vi "kvCanAccept.vi"(2 "error in (no error)":errorcluster, 3 "Accept Flag":i32(ring)=3 items=["Reserve 0", "Reserve 1", "Reserve 2", "Set Standard Code", "Set Standard Mask", "Set Extended Code", "Set Extended Mask"], 4 "Envelope Mask or Code":u32, 5 "Channel Handle (input only)":i32) -> (0 "error out":errorcluster, 1 "Channel Handle (ouput only)":i32)   [LabVIEW 2022 SP3]
doc: "This routine sets the message acceptance filters on a CAN channel."
uses:
  canlib32.dll
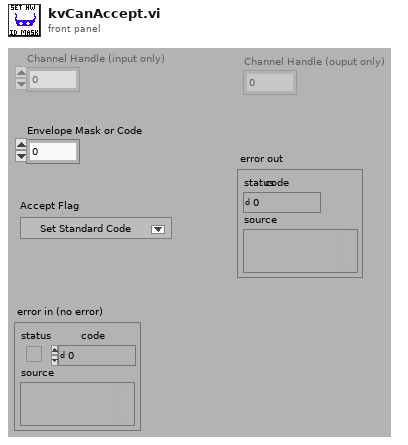
[diagram p1: front panel]
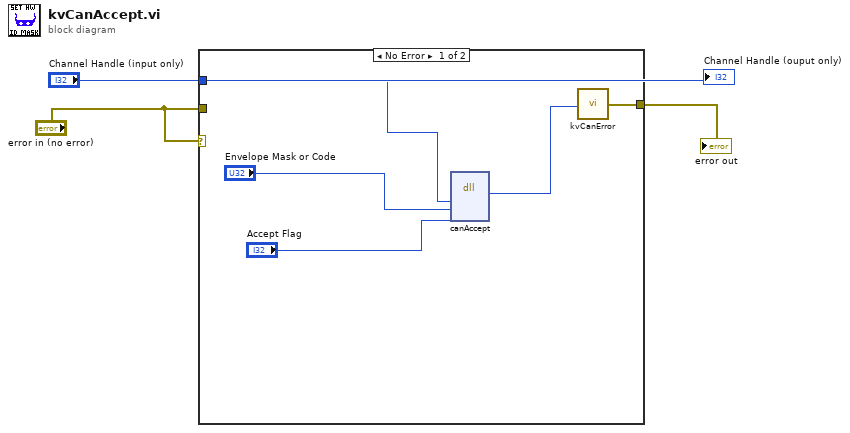
[diagram p0: block diagram]
diagram:
  n1 = case shown="No Error" "error in (no error)" {
    tunnel: [w8 w9] -> w3
    tunnel: "error in (no error)" -> [_ w9]
    tunnel: "Channel Handle (input only)" -> [w6 _]
    frame No Error {
      n2 = dll-call lib="canlib32.dll" fn="canAccept" label="Call CanAccept"("channelHandle"=w6, "envelope"="Envelope Mask or Code", "flag"="Accept Flag") -> (w7:i32)  [unwired: 6 in, 2 out]
      n3 = call "kvCanError.vi"("error code"=w7) -> ("error out"=w8:errorcluster)
    }
    frame Error {
    }
  }
  "error out" <- w3
  "Channel Handle (ouput only)" <- "Channel Handle (input only)"
